vi "niDTS BT INSTR TX Configure TXP.vi"(8 "error in (no error)":errorcluster, 11 "niDTS BT INSTR TX in":refnum<class "niDTS BT INSTR TX.lvclass">) -> (0 "error out":errorcluster, 3 "niDTS BT INSTR TX out":refnum<class "niDTS BT INSTR TX.lvclass">)   [LabVIEW 2015, in "niDTS BT.lvlib" / "niDTS BT INSTR TX.lvclass"]
doc: "Sets:\n\n* TriggerThreshold\n* Trigger Source\n* MinQuietTimeDuration\n* TriggerTimeout"
uses:
  niDTS BT INSTR TX.lvclass
  niDTS BT INSTR TX.lvclass/niDTS BT INSTR TX.ctl
  RiviInstDriver/niRfsaBT/Objects/niRfsaBt.lvclass
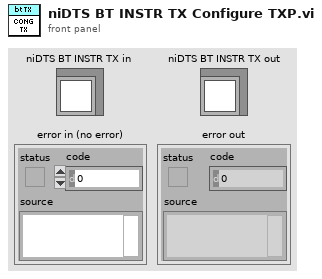
[diagram p1: front panel]
types:
  T1 = typedef "niRfsaBT.lvclass/niRfsaBT INC Handle.ctl" = refnum<data-value>
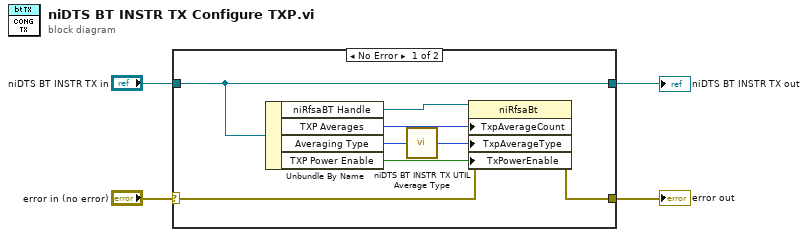
[diagram p0: block diagram]
diagram:
  n1 = case shown="No Error" "error in (no error)" {
    selector: "error in (no error)" -> [w12 w14]
    tunnel: [w11 w14] -> w3
    tunnel: "niDTS BT INSTR TX in" -> [w9 w13]
    tunnel: [w9 w13] -> w1
    frame No Error {
      n2 = Unbundle By Name(w9) -> ("niRfsaBT Handle"=w10:T1, "TXP Averages"=w7:i32, "Averaging Type"=w6:enum16{"RMS", "LOG", "SCALAR", "MAX", "MIN"}, "TXP Power Enable"=w8:bool)
      n3 = call "niDTS BT INSTR TX UTIL Average Type.vi"("Type In"=w6) -> ("Type Out"=w5:enum16{"RMS", "LOG", "SCALar", "MAX", "MIN"})  [unwired: 14 in]
      n4 = property class="niRfsaBt"(reference=w10, error in=w12, "TxpAverageCount"=w7, "TxpAverageType"=w5, "TxPowerEnable"=w8) -> (error out=w11:errorcluster)  [unwired: 1 out]
    }
    frame Error {
    }
  }
  "error out" <- w3
  "niDTS BT INSTR TX out" <- w1
